vi "MGI Button Dialog CORE.vi"(0 "Hide calling VI? (FALSE)":bool, 4 "Allow user to close window? (TRUE)":bool=TRUE, 5 "Justify Message (Left)":enum16{"Left", "Center", "Right"}(ring), 6 "Keyboard Shortcuts (Left is <Enter>)":T1={"Left Button Key Shortcut"={"Control"=FALSE, "Shift"=FALSE, "Key"="<Enter>"}, "Center Button Key Shortcut"={"Control"=FALSE, "Shift"=FALSE, "Key"=""}, "Right Button Key Shortcut"={"Control"=FALSE, "Shift"=FALSE, "Key"=""}}, 7 "Window Title (\"\")":string, 8 "Right Button Text (\"Cancel\")":string="Cancel", 9 "Center Button Text (\"No\")":string="No", 10 "Left Button Text (\"Yes\")":string="Yes", 11 "message":string) -> (2 "Left Button?":bool, 3 "Which Button?":T2(ring)=enum."Center Button")   [LabVIEW 2020]
doc: "Displays text in a dialog with three buttons. The output enum indicates which of the three buttons the user chose, or it indicates that the user closed the dialog without making any choice."
panel:
  in  "OK":string="OK"
  out "C-Message":string
  in  "Right Button":bool
  in  "Center Button":bool
  in  "Left Button":bool
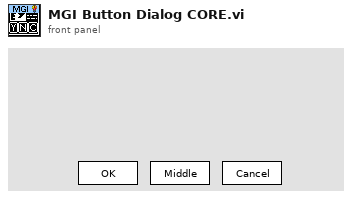
[diagram p1: front panel]
types:
  T1 = cluster{"Left Button Key Shortcut":cluster{"Control":bool, "Shift":bool, "Key":string}, "Center Button Key Shortcut":cluster{"Control":bool, "Shift":bool, "Key":string}, "Right Button Key Shortcut":cluster{"Control":bool, "Shift":bool, "Key":string}}
  T2 = enum16{"Left Button", "Center Button", "Right Button", "Window Close"}
  T3 = enum32{"Invalid", "Default", "Floating", "Floating/Auto-Hide", "Modal"}
  T4 = cluster{"left":i16, "top":i16, "right":i16, "bottom":i16}
  T5 = cluster{"Control":bool, "Shift":bool, "Key":string}
  T6 = cluster{bool, "Control":bool, "Shift":bool, "Key":string}
  T7 = typedef "LVRectTypeDef.ctl" = cluster{"Left":i16, "Top":i16, "Right":i16, "Bottom":i16}
  T8 = typedef "LVPointTypeDef.ctl" = cluster{"Horizontal":i16, "Vertical":i16}
  T9 = enum32{"Invalid", "Standard", "Closed", "Hidden", "Minimized", "Maximized"}
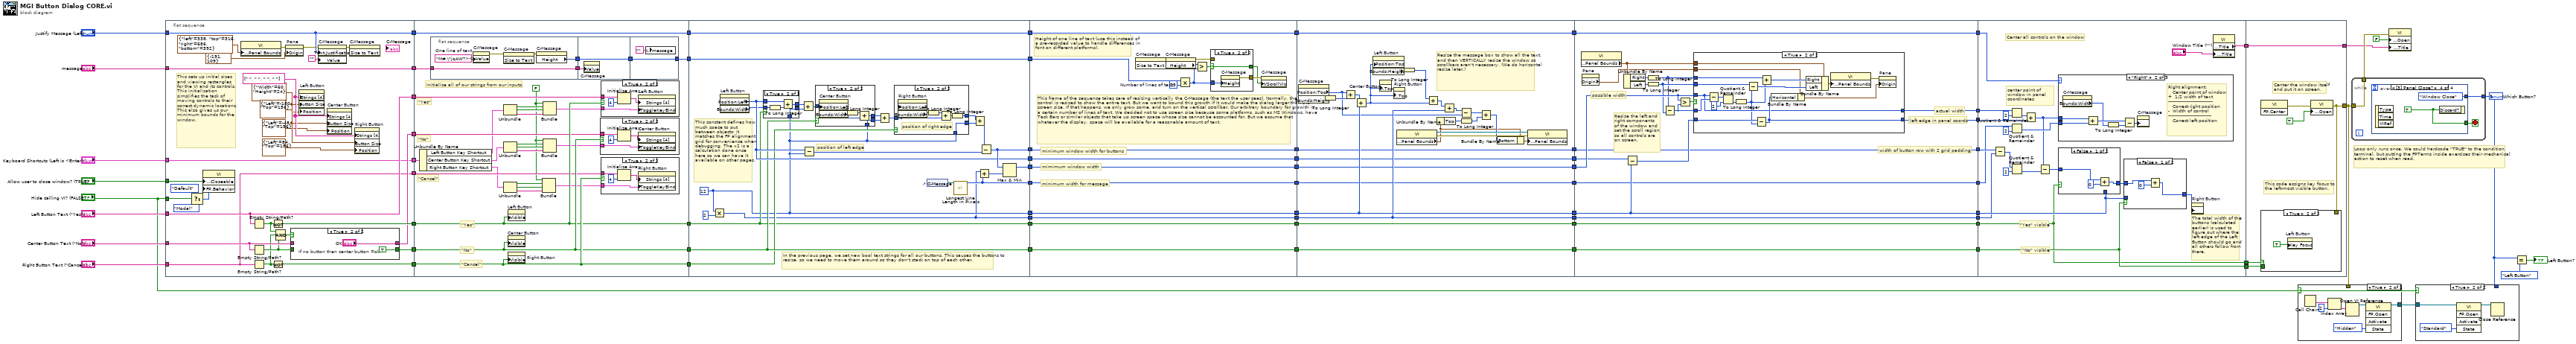
[diagram p0: block diagram]
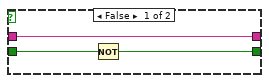
[diagram p4: hidden frame]
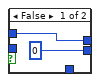
[diagram p8: hidden frame]
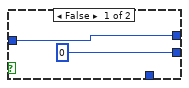
[diagram p9: hidden frame]
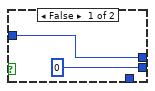
[diagram p10: hidden frame]
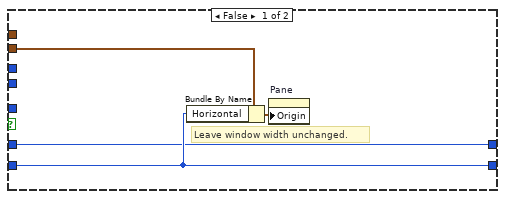
[diagram p12: hidden frame]
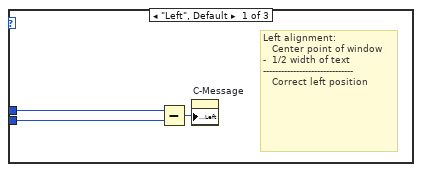
[diagram p13: hidden frame]
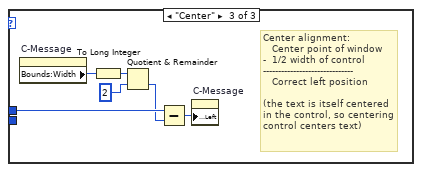
[diagram p14: hidden frame]
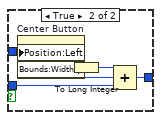
[diagram p15: hidden frame]
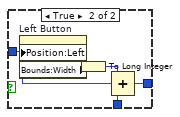
[diagram p16: hidden frame]
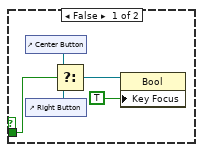
[diagram p17: hidden frame]
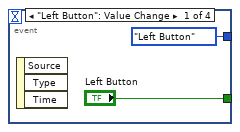
[diagram p18: hidden frame]
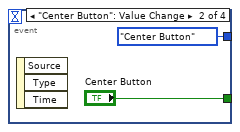
[diagram p19: hidden frame]
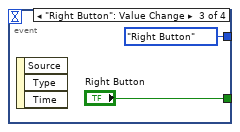
[diagram p20: hidden frame]
diagram:
  # "Loop only runs once. We could hardcode \"TRUE\" to the condition terminal, but putting the FPTerms inside exercises their mechanical action to reset when read."
  n1 = flat-sequence {
    tunnel: [w90] -> w17
    tunnel: [w92] -> w16
    tunnel: [w91] -> w15
    tunnel: [w86] -> w14
    tunnel: [w87] -> w13
    tunnel: [w84] -> w12
    tunnel: [w83] -> w11
    tunnel: "Left Button Text (\"Yes\")" -> [w86]
    tunnel: "Center Button Text (\"No\")" -> [w85]
    tunnel: "Right Button Text (\"Cancel\")" -> [w84]
    tunnel: "Justify Message (Left)" -> [w83]
    tunnel: "Keyboard Shortcuts (Left is <Enter>)" -> [w80]
    tunnel: [w80] -> w10
    tunnel: "message" -> [w79]
    tunnel: [w79] -> w9
    tunnel: "Allow user to close window? (TRUE)" -> [w78]
    tunnel: "Hide calling VI? (FALSE)" -> [w73]
    tunnel: w17 -> [w134]
    tunnel: [w134] -> w67
    tunnel: w16 -> [w133]
    tunnel: [w133] -> w66
    tunnel: w15 -> [w132]
    tunnel: [w132] -> w65
    tunnel: w14 -> [w131]
    tunnel: w13 -> [w130]
    tunnel: w12 -> [w129]
    tunnel: w11 -> [w128]
    tunnel: [w128] -> w64
    tunnel: [w124] -> w63
    tunnel: w10 -> [w127]
    tunnel: w9 -> [w123]
    tunnel: [w179] -> w62
    tunnel: [w176] -> w61
    tunnel: [w175] -> w60
    tunnel: [w157] -> w59
    tunnel: [w156] -> w58
    tunnel: w67 -> [w168]
    tunnel: w66 -> [w170]
    tunnel: [w170] -> w57
    tunnel: w65 -> [w166]
    tunnel: [w166] -> w56
    tunnel: [w161] -> w55
    tunnel: w64 -> [w160]
    tunnel: [w160] -> w54
    tunnel: w63 -> [w159]
    tunnel: [w159] -> w53
    tunnel: w62 -> [w211]
    tunnel: [w211] -> w52
    tunnel: w61 -> [w210]
    tunnel: [w210] -> w51
    tunnel: w60 -> [w209]
    tunnel: [w209] -> w50
    tunnel: w59 -> [w208]
    tunnel: [w208] -> w49
    tunnel: w58 -> [w207]
    tunnel: [w207] -> w48
    tunnel: w57 -> [w206]
    tunnel: [w206] -> w47
    tunnel: w56 -> [w205]
    tunnel: [w205] -> w46
    tunnel: w55 -> [w204]
    tunnel: [w204] -> w45
    tunnel: w54 -> [w203]
    tunnel: [w203] -> w44
    tunnel: w53 -> [w213]
    tunnel: w52 -> [w232]
    tunnel: [w232] -> w43
    tunnel: w51 -> [w231]
    tunnel: [w231] -> w42
    tunnel: w50 -> [w230]
    tunnel: [w230] -> w41
    tunnel: w49 -> [w241]
    tunnel: [w241] -> w40
    tunnel: w48 -> [w242]
    tunnel: [w242] -> w39
    tunnel: w47 -> [w229]
    tunnel: [w229] -> w38
    tunnel: w46 -> [w228]
    tunnel: [w228] -> w37
    tunnel: w45 -> [w227]
    tunnel: [w227] -> w36
    tunnel: w44 -> [w226]
    tunnel: [w226] -> w35
    tunnel: w43 -> [w270]
    tunnel: [w265] -> w34
    tunnel: w42 -> [w258]
    tunnel: [w258] -> w33
    tunnel: w41 -> [w264]
    tunnel: w40 -> [w263]
    tunnel: [w263] -> w32
    tunnel: w39 -> [w257]
    tunnel: [w257] -> w31
    tunnel: [w261] -> w30
    tunnel: w38 -> [w256]
    tunnel: [w256] -> w29
    tunnel: w37 -> [w255]
    tunnel: [w255] -> w28
    tunnel: w36 -> [w254]
    tunnel: [w254] -> w27
    tunnel: w35 -> [w253]
    tunnel: [w253] -> w26
    tunnel: [w295] -> w25
    tunnel: w34 -> [w314]
    tunnel: w33 -> [w307]
    tunnel: w32 -> [w311]
    tunnel: w31 -> [w306]
    tunnel: w30 -> [w313]
    tunnel: w29 -> [w294]
    tunnel: w28 -> [w293]
    tunnel: w27 -> [w299]
    tunnel: w26 -> [w300]
    tunnel: [w294] -> w8
    tunnel: [w293] -> w7
    tunnel: [w348] -> w1
    tunnel: [w350] -> w68
    tunnel: w25 -> [w350]
    tunnel: w8 -> [w346]
    tunnel: w7 -> [w347]
    frame #0 {
      w100 = string[] [" ", " ", " ", " "] ("Strings [4]")
      w99 = cluster{"Width":u32, "Height":u32} {"Width"=60, "Height"=24} ("Button Size")
      # "This sets up initial sizes and viewing rectangles\nfor the VI and its controls. This initialization\nsimplifies the task of moving controls to their\ncorrect dynamic locations. This also gives us our\nminimum bounds for the window."
      n2 = Select(t=T3."Default" ("Front Panel Window:Behavior"), s=w73, f=T3."Modal" ("Front Panel Window:Behavior")) -> (s? t:f=w74:T3)
      n3 = property class="VI"("Front Panel Window:Closeable"=w78, "FP.Behavior"=w74) -> ()  [unwired: 2 in, 2 out]
      n4 = property class="VI"("Front Panel Window:Panel Bounds"=T4 {"left"=338, "top"=316, "right"=686, "bottom"=392} ("Front Panel.PanelBounds")) -> (error out=w77:errorcluster)  [unwired: 2 in, 1 out]
      n5 = Empty String/Path?(string/path=w86) -> (empty?=w94:bool)
      n6 = Empty String/Path?(string/path=w85) -> (empty?=w82:bool)
      n7 = Empty String/Path?(string/path=w84) -> (empty?=w81:bool)
      n8 = Not(x=w94) -> (.not. x?=w91:bool)
      n9 = Not(x=w81) -> (.not. x?=w90:bool)
      n10 = Compound Arithmetic op=AND(w94, w81, w82) -> (w93:bool)
      n11 = property on="Pane" class="Pane"(error in=w77, "Origin"=cluster{"Horizontal":i16, "Vertical":i16} {"Horizontal"=-191, "Vertical"=109} ("Front Panel.Origin")) -> (error out=w76:errorcluster)  [unwired: 1 in, 1 out]
      n12 = case shown="True" w93 {
        tunnel: w82 -> [w103 _]
        tunnel: [w102 TRUE] -> w92
        tunnel: w85 -> [w101 _]
        tunnel: [w101 "OK"] -> w87
        frame False {
          n13 = Not(x=w103) -> (.not. x?=w102:bool)
        }
        frame True {
          # "If no button then center button =ok"
        }
      }
      n14 = property on="Left Button" class="Bool"("Strings [4]"=w100, "Button Size"=w99, "Position"=cluster{"Left":i32, "Top":i32} {"Left"=-180, "Top"=156}) -> ()  [unwired: 2 in, 2 out]
      n15 = property on="C-Message" class="Str"(error in=w76, "Text.Justification"=w83, "Value"="") -> (error out=w95:errorcluster)  [unwired: 1 in, 1 out]
      n16 = property on="Center Button" class="Bool"("Strings [4]"=w100, "Button Size"=w99, "Position"=cluster{"Left":i32, "Top":i32} {"Left"=-48, "Top"=156}) -> ()  [unwired: 2 in, 2 out]
      n17 = invoke on="C-Message" class="Str" method="Size to Text"(error in=w95) -> ()  [unwired: 2 in, 3 out]
      n18 = property on="Right Button" class="Bool"("Strings [4]"=w100, "Button Size"=w99, "Position"=cluster{"Left":i32, "Top":i32} {"Left"=84, "Top"=156}) -> ()  [unwired: 2 in, 2 out]
    }
    frame #1 {
      w108 = FALSE
      # "\"Cancel\""
      # "\"No\""
      # "\"Yes\""
      # "\"Cancel\""
      # "\"No\""
      # "\"Yes\""
      # "Initialize all of our strings from our inputs."
      n19 = Unbundle By Name(w127) -> ("Left Button Key Shortcut"=w121:T5, "Center Button Key Shortcut"=w113:T5, "Right Button Key Shortcut"=w107:T5)
      n20 = flat-sequence {
        tunnel: [w136] -> w126
        tunnel: w123 -> [w135]
        tunnel: [w135] -> w122
        tunnel: w126 -> [w141]
        tunnel: [w141] -> w125
        tunnel: w122 -> [w140]
        tunnel: w125 -> [w142]
        tunnel: [w142] -> w124
        frame #0 {
          w139 = "M#,\"jqAW?><"  # One line of text
          n21 = property on="C-Message" class="Str"("Value"=w139) -> (error out=w137:errorcluster)  [unwired: 2 in, 1 out]
          n22 = invoke on="C-Message" class="Str" method="Size to Text"(error in=w137) -> (error out=w138:errorcluster)  [unwired: 2 in, 2 out]
          n23 = property on="C-Message" class="Str"(error in=w138) -> ("Height"=w136:u32)  [unwired: 1 in, 2 out]
        }
        frame #1 {
          n24 = property on="C-Message" class="Str"("Value"=w140) -> ()  [unwired: 2 in, 2 out]
        }
        frame #2 {
          n25 = local write "message"("") -> ()
        }
      }
      n26 = Unbundle(w121) -> ("Control"=w120:bool, "Shift"=w119:bool, "Key"=w118:string)
      n27 = Unbundle(w113) -> ("Control"=w116:bool, "Shift"=w115:bool, "Key"=w114:string)
      n28 = Unbundle(w107) -> ("Control"=w111:bool, "Shift"=w110:bool, "Key"=w109:string)
      n29 = property on="Left Button" class="Bool"("Visible"=w132) -> ()  [unwired: 2 in, 2 out]
      n30 = property on="Center Button" class="Bool"("Visible"=w133) -> ()  [unwired: 2 in, 2 out]
      n31 = property on="Right Button" class="Bool"("Visible"=w134) -> ()  [unwired: 2 in, 2 out]
      n32 = Bundle(w108, "Control"=w111, "Shift"=w110, "Key"=w109) -> (w106:T6)  [unwired: 1 in]
      n33 = Bundle(w108, "Control"=w120, "Shift"=w119, "Key"=w118) -> (w117:T6)  [unwired: 1 in]
      n34 = Bundle(w108, "Control"=w116, "Shift"=w115, "Key"=w114) -> (w112:T6)  [unwired: 1 in]
      n35 = case shown="True" w133 {
        tunnel: w112 -> [_ w149]
        tunnel: w130 -> [_ w148]
        frame False {
        }
        frame True {
          n36 = Initialize Array(w148, 4 ("dimension size")) -> (w151:string[])
          n37 = property on="Center Button" class="Bool"("Strings [4]"=w151, "ToggleKeyBind"=w149) -> ()  [unwired: 2 in, 2 out]
        }
      }
      n38 = case shown="True" w132 {
        tunnel: w131 -> [_ w153]
        tunnel: w117 -> [_ w152]
        frame False {
        }
        frame True {
          n39 = Initialize Array(w153, 4 ("dimension size")) -> (w155:string[])
          n40 = property on="Left Button" class="Bool"("Strings [4]"=w155, "ToggleKeyBind"=w152) -> ()  [unwired: 2 in, 2 out]
        }
      }
      n41 = case shown="True" w134 {
        tunnel: w106 -> [_ w145]
        tunnel: w129 -> [_ w144]
        frame False {
        }
        frame True {
          n42 = Initialize Array(w144, 4 ("dimension size")) -> (w147:string[])
          n43 = property on="Right Button" class="Bool"("Strings [4]"=w147, "ToggleKeyBind"=w145) -> ()  [unwired: 2 in, 2 out]
        }
      }
    }
    frame #2 {
      w157 = 12 ("grid spacing")
      # "This constant defines how much space to put between objects; it matches the FP alignment grid for convenience when debugging. The x2 is a calculation done once here so we can have it available on other pages."
      # "In the previous page, we set new bool text strings for all our buttons. This causes the buttons to resize, so we need to move them around so they don't stack on top of each other."
      # "position of left edge"
      n44 = Multiply(x=w157, y=2) -> (x*y=w156:i32)
      n45 = property on="Left Button" class="Bool"() -> ("Position:Left"=w175:i32, "Bounds:Width"=w172:u32)  [unwired: 2 in, 2 out]
      n46 = case shown="True" w166 {
        tunnel: w175 -> [w182 w187]
        tunnel: w172 -> [_ w186]
        tunnel: [w182 w185] -> w167
        tunnel: w157 -> [_ w183]
        tunnel: [0 w183] -> w165
        frame False {
        }
        frame True {
          n47 = To Long Integer(number=w186) -> (32bit integer=w184:i32)
          n48 = Add(x=w187, y=w184) -> (x+y=w185:i32)
        }
      }
      n49 = Add(x=w167, y=w165) -> (x+y=w173:i32)
      n50 = Subtract(x=w175, y=w157) -> (x-y=w177:i32)
      n51 = case shown="True" w170 {
        tunnel: w173 -> [w197 w202]
        tunnel: [w197 w201] -> w171
        tunnel: [0 w198] -> w164
        tunnel: w157 -> [_ w198]
        frame False {
        }
        frame True {
          n52 = property on="Center Button" class="Bool"("Position:Left"=w202) -> ("Bounds:Width"=w200:u32)  [unwired: 2 in, 2 out]
          n53 = To Long Integer(number=w200) -> (32bit integer=w199:i32)
          n54 = Add(x=w199, y=w202) -> (x+y=w201:i32)
        }
      }
      n55 = Add(x=w171, y=w164) -> (x+y=w174:i32)
      n56 = case shown="True" w168 {
        tunnel: w174 -> [w189 w195]
        tunnel: [w189 w193] -> w169
        tunnel: [0 w190] -> w163
        tunnel: w157 -> [_ w190]
        frame False {
        }
        frame True {
          # "position of right edge"
          n57 = property on="Right Button" class="Bool"("Position:Left"=w195) -> ("Bounds:Width"=w192:u32)  [unwired: 2 in, 2 out]
          n58 = To Long Integer(number=w192) -> (32bit integer=w191:i32)
          n59 = Add(x=w191, y=w195) -> (x+y=w194:i32)
          n60 = To Long Integer(number=w194) -> (32bit integer=w193:i32)
        }
      }
      n61 = control-ref of="C-Message"() -> (w162:refnum<vi>)
      n62 = call <vilib>:"Longest Line Length in Pixels.vi"("String"=w162) -> ("longest line length"=w161:i32)  [unwired: 9 in]
      n63 = Add(x=w169, y=w163) -> (x+y=w178:i32)
      n64 = Add(x=w156, y=w161) -> (x+y=w180:i32)
      n65 = Subtract(x=w178, y=w177) -> (x-y=w176:i32)
      n66 = Max & Min(x=w176, y=w180) -> (max(x,y)=w179:i32)  [unwired: 1 out]
    }
    frame #3 {
      w214 = u32 25  # Number of lines of text
      # "minimum window width for buttons"
      # "mimimum window width"
      # "minimum width for message"
      # "Height of one line of text (use this instead of a pre-recorded value to handle differences in font on different platforms)."
      # "This frame of the sequence takes care of resizing vertically the C-Message (the text the user sees). Normally, the string control is resized to show the entire text. But we want to bound this growth if it would make the dialog larger than the screen size. If that happens, we only grow some, and turn on the vertical scrollbar. Our arbitrary boundary for growith is a certain number of lines of text. We decided not to use screen size because some platforms, such as MS Windows, have Task Bars or similar objects that take up screen space whose size cannot be accounted for. But we assume that whatever the display, space will be available for a reasonable amount of text."
      n67 = invoke on="C-Message" class="Str" method="Size to Text"() -> (error out=w220:errorcluster)  [unwired: 3 in, 2 out]
      n68 = property on="C-Message" class="Str"(error in=w220) -> (error out=w215:errorcluster, "Height"=w219:u32)  [unwired: 1 in, 1 out]
      n69 = Multiply(x=w213, y=w214) -> (x*y=w212:u32)
      n70 = Greater?(x=w219, y=w212) -> (0:w218:bool)
      n71 = case shown="True" w218 {
        selector: w218 -> [w222 w224]
        tunnel: [w221 w225] -> w217
        tunnel: [w222 w224] -> w216
        tunnel: w215 -> [w221 _]
        tunnel: w212 -> [_ w223]
        frame False {
        }
        frame True {
          n72 = property on="C-Message" class="Str"("Height"=w223) -> (error out=w225:errorcluster)  [unwired: 2 in, 1 out]
        }
      }
      n73 = property on="C-Message" class="Str"(error in=w217, "VScrollVis"=w216) -> ()  [unwired: 1 in, 2 out]
    }
    frame #4 {
      # "Resize the message box to show all the text, and then VERTICALLY resize the window so scrollbars aren't necessary. (We do horizontal resize later.)"
      n74 = property on="C-Message" class="Str"() -> ("Position:Top"=w234:i32, "Bounds:Height"=w233:u32)  [unwired: 2 in, 2 out]
      n75 = To Long Integer(number=w233) -> (32bit integer=w240:i32)
      n76 = Add(x=w234, y=w240) -> (x+y=w243:i32)
      n77 = Add(x=w243, y=w241) -> (x+y=w236:i32)
      n78 = property on="Left Button" class="Bool"("Position:Top"=w236) -> ("Bounds:Height"=w237:u32)  [unwired: 2 in, 2 out]
      n79 = property on="Center Button" class="Bool"("Position:Top"=w236) -> ()  [unwired: 2 in, 2 out]
      n80 = property on="Right Button" class="Bool"("Position:Top"=w236) -> ()  [unwired: 2 in, 2 out]
      n81 = property class="VI"() -> (reference out=w249:refnum<vi>, error out=w250:errorcluster, "Front Panel Window:Panel Bounds"=w238:T7)  [unwired: 2 in]
      n82 = To Long Integer(number=w237) -> (32bit integer=w235:i32)
      n83 = Add(x=w235, y=w236) -> (x+y=w244:i32)
      n84 = Unbundle By Name(w238) -> ("Top"=w247:i16)
      n85 = Add(x=w244, y=w242) -> (x+y=w245:i32)
      n86 = Subtract(x=w245, y=w234) -> (x-y=w248:i32)
      n87 = To Long Integer(number=w247) -> (32bit integer=w239:i32)
      n88 = Add(x=w248, y=w239) -> (x+y=w246:i32)
      n89 = Bundle By Name(cluster=w238, "Bottom"=w246) -> (w251:T7)
      n90 = property class="VI"(reference=w249, error in=w250, "Front Panel Window:Panel Bounds"=w251) -> ()  [unwired: 2 out]
    }
    frame #5 {
      # "left edge in panel coords"
      # "width of button row with 2 grid padding"
      # "Resize the left and\nright components\nof the window and\nset the scroll region\nso all controls are \non screen."
      # "actual width"
      # "possible width"
      n91 = property class="VI"() -> ("Front Panel Window:Panel Bounds"=w267:T7)  [unwired: 2 in, 2 out]
      n92 = property on="Pane" class="Pane"() -> ("Origin"=w252:T8)  [unwired: 2 in, 2 out]
      n93 = Unbundle By Name(w267) -> ("Right"=w269:i16, "Left"=w268:i16)
      n94 = Subtract(x=w264, y=w263) -> (x-y=w262:i32)
      n95 = To Long Integer(number=w269) -> (32bit integer=w259:i32)
      n96 = To Long Integer(number=w268) -> (32bit integer=w260:i32)
      n97 = Subtract(x=w259, y=w260) -> (x-y=w271:i32)
      n98 = Greater?(x=w270, y=w271) -> (0:w266:bool)
      n99 = case shown="True" w266 {
        tunnel: w271 -> [w273 w292]
        tunnel: w270 -> [_ w279]
        tunnel: w259 -> [_ w287]
        tunnel: w260 -> [_ w288]
        tunnel: w267 -> [_ w289]
        tunnel: [w275 w281] -> w265
        tunnel: w252 -> [w274 w282]
        tunnel: w262 -> [w275 w280]
        tunnel: [w273 w279] -> w261
        frame False {
          # "Leave window width unchanged."
          n100 = Bundle By Name(cluster=w274, "Horizontal"=w275) -> (w272:T8)
          n101 = property on="Pane" class="Pane"("Origin"=w272) -> ()  [unwired: 2 in, 2 out]
        }
        frame True {
          n102 = Subtract(x=w279, y=w292) -> (x-y=w291:i32)
          n103 = Quotient & Remainder(x=w291, y=2) -> (floor(x/y)=w284:i32)  [unwired: 1 out]
          n104 = To Long Integer(number=w284) -> (32bit integer=w278:i32)
          n105 = Subtract(x=w288, y=w278) -> (x-y=w285:i32)
          n106 = Subtract(x=w280, y=w278) -> (x-y=w281:i32)
          n107 = Add(x=w287, y=w278) -> (x+y=w286:i32)
          n108 = Bundle By Name(cluster=w282, "Horizontal"=w281) -> (w276:T8)
          n109 = Bundle By Name(cluster=w289, "Right"=w286, "Left"=w285) -> (w283:T7)
          n110 = property class="VI"("Front Panel Window:Panel Bounds"=w283) -> (error out=w277:errorcluster)  [unwired: 2 in, 1 out]
          n111 = property on="Pane" class="Pane"(error in=w277, "Origin"=w276) -> ()  [unwired: 1 in, 2 out]
        }
      }
    }
    frame #6 {
      # "\"No\" visible"
      # "\"Yes\" visible"
      # "The total width of the buttons (calculated earlier) is used to figure out where the left edge of the Left Button should go and all others follow from there."
      # "center point of window in panel coordinates"
      # "Center all controls on the window"
      n112 = Subtract(x=w307, y=w306) -> (x-y=w308:i32)
      n113 = Quotient & Remainder(x=w313, y=2) -> (floor(x/y)=w310:i32)  [unwired: 1 out]
      n114 = Quotient & Remainder(x=w299, y=2) -> (floor(x/y)=w298:i32)  [unwired: 1 out]
      n115 = Quotient & Remainder(x=w308, y=2) -> (floor(x/y)=w305:i32)  [unwired: 1 out]
      n116 = Add(x=w310, y=w314) -> (x+y=w297:i32)
      n117 = Subtract(x=w297, y=w305) -> (x-y=w304:i32)
      n118 = case shown="\"Right\"" w300 {
        tunnel: w297 -> [w317 w323 w325]
        tunnel: w298 -> [w315 w322 _]
        frame "Left", Default {
          # "Left alignment:\n   Center point of window\n-  1/2 width of text\n------------------------------\n   Correct left position"
          n119 = Subtract(x=w317, y=w315) -> (x-y=w316:i32)
          n120 = property on="C-Message" class="Str"("Position:Left"=w316) -> ()  [unwired: 2 in, 2 out]
        }
        frame "Right" {
          # "Right alignment:\n   Center point of window\n+  1/2 width of text\n------------------------------\n   Correct right position\n-  Width of control\n-----------------------------\n   Correct left position"
          n121 = property on="C-Message" class="Str"() -> ("Bounds:Width"=w319:u32)  [unwired: 2 in, 2 out]
          n122 = Add(x=w323, y=w322) -> (x+y=w321:i32)
          n123 = To Long Integer(number=w319) -> (32bit integer=w318:i32)
          n124 = Subtract(x=w321, y=w318) -> (x-y=w320:i32)
          n125 = property on="C-Message" class="Str"("Position:Left"=w320) -> ()  [unwired: 2 in, 2 out]
        }
        frame "Center" {
          # "Center alignment:\n   Center point of window\n-  1/2 width of control\n------------------------------\n   Correct left position\n\n(the text is itself centered in the control, so centering control centers text)"
          n126 = property on="C-Message" class="Str"() -> ("Bounds:Width"=w328:u32)  [unwired: 2 in, 2 out]
          n127 = To Long Integer(number=w328) -> (32bit integer=w326:i32)
          n128 = Quotient & Remainder(x=w326, y=2) -> (floor(x/y)=w324:i32)  [unwired: 1 out]
          n129 = Subtract(x=w325, y=w324) -> (x-y=w327:i32)
          n130 = property on="C-Message" class="Str"("Position:Left"=w327) -> ()  [unwired: 2 in, 2 out]
        }
      }
      n131 = case shown="False" w293 {
        tunnel: w311 -> [_ w345]
        tunnel: w304 -> [w340 w344]
        tunnel: [w339 w342] -> w303
        frame False {
          n132 = Add(x=w340, y=0) -> (x+y=w339:i32)
        }
        frame True {
          n133 = property on="Left Button" class="Bool"("Position:Left"=w344) -> ("Bounds:Width"=w343:u32)  [unwired: 2 in, 2 out]
          n134 = To Long Integer(number=w343) -> (32bit integer=w341:i32)
          n135 = Compound Arithmetic op=ADD(w341, w344, w345) -> (w342:i32)
        }
      }
      n136 = case shown="False" w294 {
        tunnel: w311 -> [_ w337]
        tunnel: w303 -> [w332 w335]
        tunnel: [w331 w334] -> w302
        frame False {
          n137 = Add(x=w332, y=0) -> (x+y=w331:i32)
        }
        frame True {
          n138 = property on="Center Button" class="Bool"("Position:Left"=w335) -> ("Bounds:Width"=w336:u32)  [unwired: 2 in, 2 out]
          n139 = To Long Integer(number=w336) -> (32bit integer=w333:i32)
          n140 = Compound Arithmetic op=ADD(w333, w335, w337) -> (w334:i32)
        }
      }
      n141 = property on="Right Button" class="Bool"("Position:Left"=w302) -> ()  [unwired: 2 in, 2 out]
      n142 = property class="VI"("Front Panel Window:Title"="Window Title (\"\")") -> ("Front Panel Window:Title"=w295:string)  [unwired: 2 in, 2 out]
    }
    frame #7 {
      # "This code assigns key focus to\nthe left-most visible button."
      # "Center the window itself and put it on screen."
      n143 = invoke class="VI" method="FP.Center"() -> (error out=w349:errorcluster)  [unwired: 3 in, 2 out]
      n144 = property class="VI"(error in=w349, "Front Panel Window:Open"=TRUE) -> (error out=w348:errorcluster)  [unwired: 1 in, 1 out]
      n145 = case shown="True" w347 {
        tunnel: w348 -> [_ _]
        tunnel: w346 -> [w356 _]
        frame False {
          n146 = control-ref of="Center Button"() -> (w355:refnum<vi>)
          n147 = control-ref of="Right Button"() -> (w354:refnum<vi>)
          n148 = Select(t=w355, s=w356, f=w354) -> (s? t:f=w353:refnum<vi>)
          n149 = property class="Bool"(reference=w353, "Key Focus"=TRUE) -> ()  [unwired: 1 in, 2 out]
        }
        frame True {
          n150 = property on="Left Button" class="Bool"("Key Focus"=TRUE) -> ()  [unwired: 2 in, 2 out]
        }
      }
    }
  }
  n151 = case shown="True" "Hide calling VI? (FALSE)" {
    tunnel: [_ w358] -> w5
    tunnel: w1 -> [_ _]
    frame False {
    }
    frame True {
      n152 = Call Chain() -> (call chain=w363:string[])
      n153 = Index Array(array=w363, index=2) -> (element=w361:string)
      n154 = Open VI Reference(vi path=w361) -> (vi reference=w360:refnum<vi>)  [unwired: 5 in, 1 out]
      n155 = invoke class="VI" method="FP.Open"(reference=w360, "State"=T9."Hidden") -> (reference out=w358:refnum<vi>)  [unwired: 3 in, 4 out]
    }
  }
  n156 = while {
    tunnel: [w366] -> w3
    tunnel: [w365] -> w69
    tunnel: w1 -> [w365]
    stop <- w364 stop-if-true
    n157 = event shown="[3] Panel Close?" {
      selector: _ -> [_ _ _ _]
      dyn-events: _ -> [_ _ _ _]
      timeout: _ -> [_ _ _ _]
      tunnel: ["Left Button" "Center Button" "Right Button" w373] -> w364
      tunnel: [T2."Left Button" ("Which Button?") T2."Center Button" ("Which Button?") T2."Right Button" ("Which Button?") T2."Window Close" ("Which Button?")] -> w366
      event "Left Button": Value Change {
        n158 = event-data() -> ()  [unwired: 1 in, 3 out]
      }
      event "Center Button": Value Change {
        n159 = event-data() -> ()  [unwired: 1 in, 3 out]
      }
      event "Right Button": Value Change {
        n160 = event-data() -> ()  [unwired: 1 in, 3 out]
      }
      event Panel Close? {
        w373 = TRUE ("Discard?")
        n161 = event-data() -> ()  [unwired: 1 in, 3 out]
        n162 = event-data("Discard?"=w373) -> ()  [unwired: 1 in, 1 out]
      }
    }
  }
  "Which Button?" <- w3
  n163 = property class="VI"(error in=w69, "Front Panel Window:Open"=FALSE, "Front Panel Window:Title"=w68) -> ()  [unwired: 1 in, 2 out]
  n164 = case shown="True" "Hide calling VI? (FALSE)" {
    tunnel: w5 -> [_ w376]
    tunnel: w3 -> [_ _]
    frame False {
    }
    frame True {
      n165 = invoke class="VI" method="FP.Open"(reference=w376, "State"=T9."Standard") -> (reference out=w375:refnum<vi>)  [unwired: 3 in, 4 out]
      n166 = Close Reference(reference=w375) -> ()  [unwired: 1 in, 1 out]
    }
  }
  n167 = Equal?(x=w3, y=T2."Left Button" ("Which Button?")) -> (x = y?=→"Left Button?":bool)
